vi "AlgorithmCentralGoal2Copy.vi"(0 "MatchBallX":dbl, 1 "MatchBallY":dbl, 2 "D1 X COM":dbl, 3 "D1Y COM":dbl, 4 "D2 X COM":dbl, 5 "D2 Y COM":dbl) -> (9 "LW":cluster{"kLW":dbl, "CoLW":dbl, "y":dbl, "y":dbl}, 11 "RW":cluster{"kRW":dbl, "CoRW":dbl, "y":dbl, "y":dbl}, 13 "output cluster":T1, 14 "Theta LG,LW":dbl, 15 "aRW":dbl, 16 "aS":dbl, 17 "min x":dbl, 18 "min x2":dbl, 19 "min x3":dbl)   [LabVIEW 2014]
panel:
  out "xD2BotS":dbl
  out "xD2ComS":dbl
  out "xD1BotS":dbl
  out "xD1ComS":dbl
  out "xD2BotR":dbl
  out "xD2ComR":dbl
  out "xD1BotR":dbl
  out "xD1ComR":dbl
  out "D2 X Bot fit 2":dbl
  out "D2 X Com fit":dbl
  out "D1 X Bot fit":dbl
  out "D1 X Com fit":dbl
  # "LOGIC"
  # "Left Goal"
  # "STRAIGHT"
  # "Left wall"
  # "Right Wall"
  # "Straight"
  # "sending data"
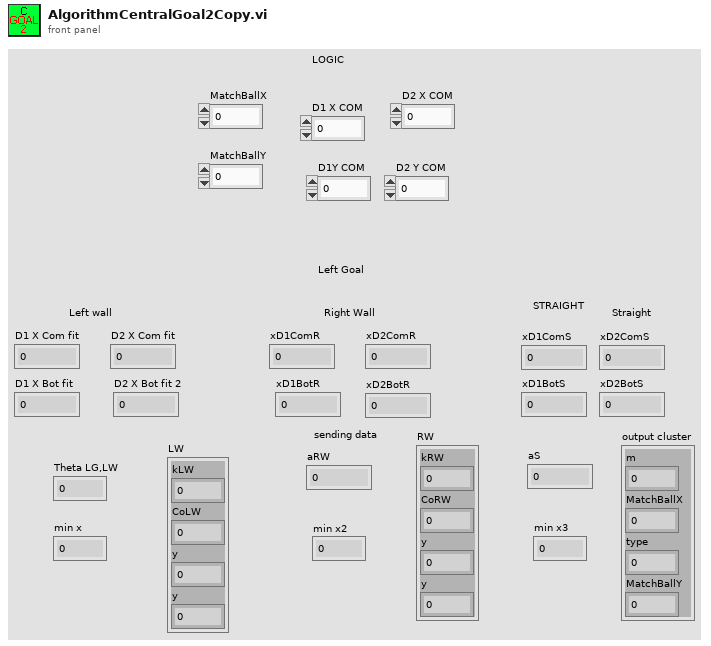
[diagram p1: front panel]
types:
  T1 = cluster{"m":dbl, "MatchBallX":dbl, "type":dbl, "MatchBallY":dbl}
  T2 = cluster{"m":dbl, "MatchBallX":dbl, "y":dbl, "MatchBallY":dbl}
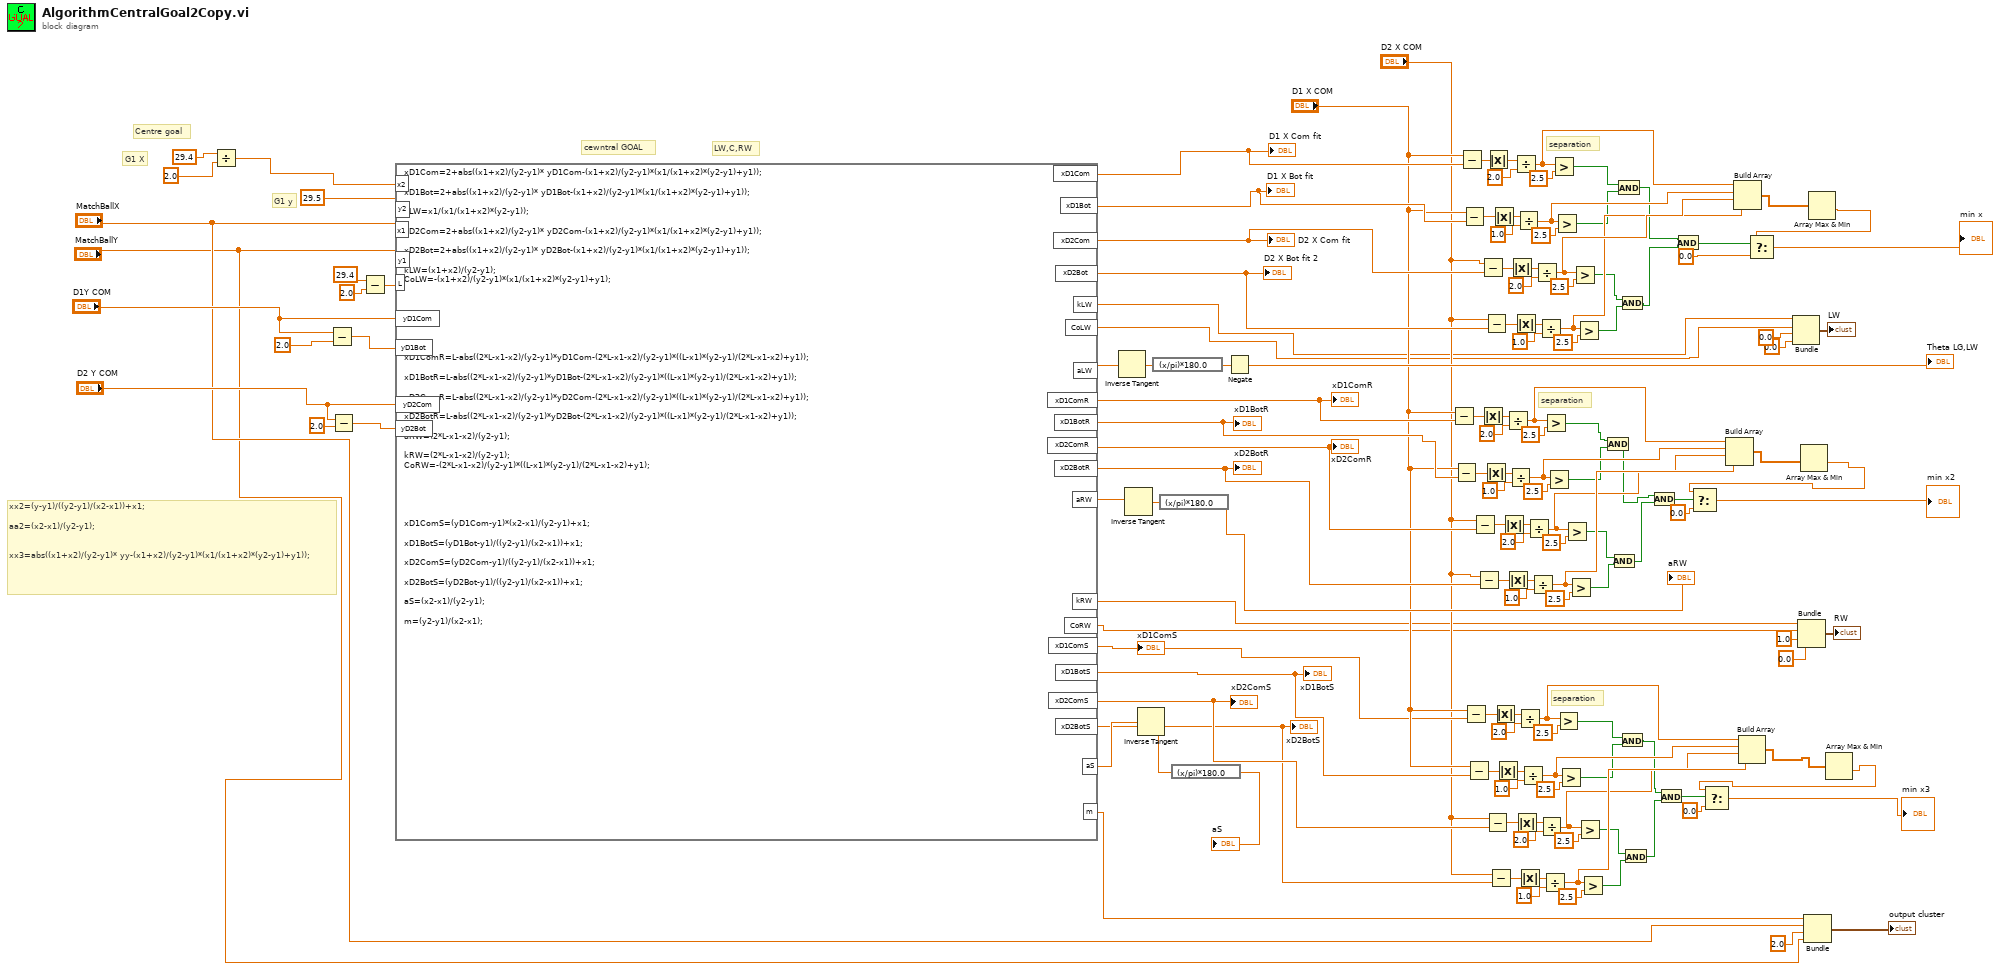
[diagram p0: block diagram]
diagram:
  # "Centre goal"
  # "G1 X"
  # "LW,C,RW"
  # "separation"
  # "separation"
  # "separation"
  # "cewntral GOAL"
  # "xx2=(y-y1)/((y2-y1)/(x2-x1))+x1;\n\naa2=(x2-x1)/(y2-y1);\n\n\nxx3=abs((x1+x2)/(y2-y1)* yy-(x1+x2)/(y2-y1)*(x1/(x1+x2)*(y2-y1)+y1));"
  # "G1 y"
  n1 = Divide(x=29.4, y=2.0) -> (x/y=w5:dbl)
  n2 = Subtract(x="D1Y COM", y=2.0) -> (x-y=w140:dbl)
  n3 = Subtract(x="D2 Y COM", y=2.0) -> (x-y=w135:dbl)
  n4 = Subtract(x=29.4 ("input variable"), y=2.0) -> (x-y=w20:dbl)
  n5 = formula code="xD1Com=2+abs((x1+x2)/(y2-y1)* yD1Com-(x1+x2)/(y2-y1)*(x1/(x1+x2)*(y2-y1)+y1));\n\nxD1Bot=2+abs((x1+x2)/(y2-y1)* yD1Bot-(x1+x2)/(y2-y1)*(x1/(x1+x2)*(y2-y1)+y1));\n\naLW=x1/(x1/(x1+x2)*(y2-y1));\n\nxD2Com=2+abs((x1+x2)/(y2-y1)* yD2Com-(x1+x2)/(y2-y1)*(x1/(x1+x2)*(y2-y1)+y1));\n\nxD2Bot=2+abs((x1+x2)/(y2-y1)* yD2Bot-(x1+x2)/(y2-y1)*(x1/(x1+x2)*(y2-y1)+y1));\n\nkLW=(x1+x2)/(y2-y1);\nCoLW=-(x1+x2)/(y2-y1)*(x1/(x1+x2)*(y2-y1)+y1);\n\n\n\n\n\n\n\nxD1ComR=L-abs((2*L-x1-x2)/(y2-y1)*yD1Com-(2*L-x1-x2)/(y2-y1)*((L-x1)*(y2-y1)/(2*L-x1-x2)+y1));\n\nxD1BotR=L-abs((2*L-x1-x2)/(y2-y1)*yD1Bot-(2*L-x1-x2)/(y2-y1)*((L-x1)*(y2-y1)/(2*L-x1-x2)+y1));\n\nxD2ComR=L-abs((2*L-x1-x2)/(y2-y1)*yD2Com-(2*L-x1-x2)/(y2-y1)*((L-x1)*(y2-y1)/(2*L-x1-x2)+y1));\n\nxD2BotR=L-abs((2*L-x1-x2)/(y2-y1)*yD2Bot-(2*L-x1-x2)/(y2-y1)*((L-x1)*(y2-y1)/(2*L-x1-x2)+y1));\n\naRW=(2*L-x1-x2)/(y2-y1);\n\nkRW=(2*L-x1-x2)/(y2-y1);\nCoRW=-(2*L-x1-x2)/(y2-y1)*((L-x1)*(y2-y1)/(2*L-x1-x2)+y1);\n\n\n\n\n\nxD1ComS=(yD1Com-y1)*(x2-x1)/(y2-y1)+x1;\n\nxD1BotS=(yD1Bot-y1)/((y2-y1)/(x2-x1))+x1;\n\nxD2ComS=(yD2Com-y1)/((y2-y1)/(x2-x1))+x1;\n\nxD2BotS=(yD2Bot-y1)/((y2-y1)/(x2-x1))+x1;\n\naS=(x2-x1)/(y2-y1);\n\nm=(y2-y1)/(x2-x1);"("x1"="MatchBallX", "x2"=w5, "y2"=29.5, "y1"="MatchBallY", "yD1Com"="D1Y COM", "yD2Com"="D2 Y COM", "yD1Bot"=w140, "yD2Bot"=w135, "L"=w20) -> ("xD1Com"=w128:dbl, "aLW"=w143:dbl, "xD1Bot"=w114:dbl, "xD2Com"=w119:dbl, "xD2Bot"=w109:dbl, "xD1ComR"=w82:dbl, "xD1BotR"=w81:dbl, "xD2ComR"=w80:dbl, "xD2BotR"=w79:dbl, "aRW"=w133:dbl, "xD1ComS"=w56:dbl, "aS"=w129:dbl, "xD1BotS"=w55:dbl, "xD2BotS"=w53:dbl, "xD2ComS"=w54:dbl, "kLW"=w18:dbl, "CoLW"=w17:dbl, "kRW"=w15:dbl, "CoRW"=w14:dbl, "m"=w12:dbl)
  "D1 X Com fit" <- w128
  "D1 X Bot fit" <- w114
  "D2 X Com fit" <- w119
  "D2 X Bot fit 2" <- w109
  "xD1ComR" <- w82
  "xD1BotR" <- w81
  "xD2ComR" <- w80
  "xD2BotR" <- w79
  "xD1ComS" <- w56
  "xD1BotS" <- w55
  "xD2ComS" <- w54
  "xD2BotS" <- w53
  n6 = Inverse Tangent(1:w143) -> (0:w144:dbl)
  n7 = Inverse Tangent(1:w133) -> (0:w134:dbl)
  n8 = Inverse Tangent(1:w129) -> (0:w130:dbl)
  n9 = expression code="(x/pi)*180.0" ("radians to degrees")(w144) -> (w141:dbl)
  n10 = expression code="(x/pi)*180.0" ("radians to degrees")(w134) -> (→"aRW":dbl)
  n11 = expression code="(x/pi)*180.0" ("radians to degrees")(w130) -> (→"aS":dbl)
  n12 = Negate(x=w141) -> (-x=→"Theta LG,LW":dbl)
  n13 = Subtract(x="D1 X COM", y=w82) -> (x-y=w83:dbl)
  n14 = Subtract(x="D1 X COM", y=w81) -> (x-y=w94:dbl)
  n15 = Subtract(x="D1 X COM", y=w128) -> (x-y=w127:dbl)
  n16 = Subtract(x="D1 X COM", y=w114) -> (x-y=w115:dbl)
  n17 = Subtract(x="D1 X COM", y=w56) -> (x-y=w58:dbl)
  n18 = Subtract(x="D1 X COM", y=w55) -> (x-y=w69:dbl)
  n19 = Subtract(x="D2 X COM", y=w80) -> (x-y=w90:dbl)
  n20 = Subtract(x="D2 X COM", y=w79) -> (x-y=w95:dbl)
  n21 = Subtract(x="D2 X COM", y=w119) -> (x-y=w120:dbl)
  n22 = Absolute Value(x=w83) -> (abs(x)=w84:dbl)
  n23 = Absolute Value(x=w94) -> (abs(x)=w93:dbl)
  n24 = Subtract(x="D2 X COM", y=w109) -> (x-y=w113:dbl)
  n25 = Subtract(x="D2 X COM", y=w54) -> (x-y=w65:dbl)
  n26 = Absolute Value(x=w127) -> (abs(x)=w126:dbl)
  n27 = Subtract(x="D2 X COM", y=w53) -> (x-y=w70:dbl)
  n28 = Absolute Value(x=w115) -> (abs(x)=w116:dbl)
  n29 = Absolute Value(x=w58) -> (abs(x)=w59:dbl)
  n30 = Absolute Value(x=w69) -> (abs(x)=w68:dbl)
  n31 = Absolute Value(x=w90) -> (abs(x)=w89:dbl)
  n32 = Divide(x=w84, y=2.0) -> (x/y=w100:dbl)
  n33 = Absolute Value(x=w95) -> (abs(x)=w96:dbl)
  n34 = Divide(x=w93, y=1.0) -> (x/y=w101:dbl)
  n35 = Absolute Value(x=w120) -> (abs(x)=w121:dbl)
  n36 = Divide(x=w126, y=2.0) -> (x/y=w107:dbl)
  n37 = Absolute Value(x=w113) -> (abs(x)=w112:dbl)
  n38 = Absolute Value(x=w65) -> (abs(x)=w64:dbl)
  n39 = Divide(x=w116, y=1.0) -> (x/y=w106:dbl)
  n40 = Divide(x=w59, y=2.0) -> (x/y=w75:dbl)
  n41 = Absolute Value(x=w70) -> (abs(x)=w71:dbl)
  n42 = Divide(x=w68, y=1.0) -> (x/y=w76:dbl)
  n43 = Divide(x=w89, y=2.0) -> (x/y=w102:dbl)
  n44 = Divide(x=w96, y=1.0) -> (x/y=w103:dbl)
  n45 = Divide(x=w121, y=2.0) -> (x/y=w105:dbl)
  n46 = Divide(x=w112, y=1.0) -> (x/y=w104:dbl)
  n47 = Divide(x=w64, y=2.0) -> (x/y=w77:dbl)
  n48 = Divide(x=w71, y=1.0) -> (x/y=w78:dbl)
  n49 = Greater?(x=w100, y=2.5) -> (0:w39:bool)
  n50 = Greater?(x=w101, y=2.5) -> (0:w38:bool)
  n51 = Greater?(x=w107, y=2.5) -> (0:w44:bool)
  n52 = Greater?(x=w106, y=2.5) -> (0:w43:bool)
  n53 = Greater?(x=w75, y=2.5) -> (0:w34:bool)
  n54 = Greater?(x=w76, y=2.5) -> (0:w33:bool)
  n55 = Greater?(x=w102, y=2.5) -> (0:w37:bool)
  n56 = Greater?(x=w103, y=2.5) -> (0:w36:bool)
  n57 = Greater?(x=w105, y=2.5) -> (0:w48:bool)
  n58 = Greater?(x=w104, y=2.5) -> (0:w47:bool)
  n59 = Greater?(x=w77, y=2.5) -> (0:w31:bool)
  n60 = Greater?(x=w78, y=2.5) -> (0:w30:bool)
  n61 = And(x=w39, y=w38) -> (x .and. y?=w40:bool)
  n62 = And(x=w37, y=w36) -> (x .and. y?=w35:bool)
  n63 = And(x=w44, y=w43) -> (x .and. y?=w42:bool)
  n64 = And(x=w48, y=w47) -> (x .and. y?=w45:bool)
  n65 = And(x=w34, y=w33) -> (x .and. y?=w32:bool)
  n66 = And(x=w31, y=w30) -> (x .and. y?=w29:bool)
  n67 = And(x=w40, y=w35) -> (x .and. y?=w41:bool)
  n68 = And(x=w32, y=w29) -> (x .and. y?=w28:bool)
  n69 = And(x=w42, y=w45) -> (x .and. y?=w46:bool)
  n70 = Build Array(w100, w101, w102, w103) -> (w25:dbl[])
  n71 = Build Array(w107, w106, w105, w104) -> (w27:dbl[])
  n72 = Build Array(w75, w76, w77, w78) -> (w23:dbl[])
  n73 = Bundle("kLW"=w18, "CoLW"=w17, "y"=0.0, "y"=0.0) -> (→"LW":cluster{"kLW":dbl, "CoLW":dbl, "y":dbl, "y":dbl})  [unwired: 1 in]
  n74 = Bundle("kRW"=w15, "CoRW"=w14, "y"=1.0, "y"=0.0) -> (→"RW":cluster{"kRW":dbl, "CoRW":dbl, "y":dbl, "y":dbl})  [unwired: 1 in]
  n75 = Array Max & Min(array=w25) -> (min value=w24:dbl)  [unwired: 3 out]
  n76 = Select(t=w24, s=w41, f=0.0 ("y")) -> (s? t:f=→"min x2":dbl)
  n77 = Bundle("m"=w12, "MatchBallX"="MatchBallX", "y"=2.0, "MatchBallY"="MatchBallY") -> (→"output cluster":T2)  [unwired: 1 in]
  n78 = Array Max & Min(array=w27) -> (min value=w26:dbl)  [unwired: 3 out]
  n79 = Select(t=w26, s=w46, f=0.0 ("y")) -> (s? t:f=→"min x":dbl)
  n80 = Array Max & Min(array=w23) -> (min value=w22:dbl)  [unwired: 3 out]
  n81 = Select(t=w22, s=w28, f=0.0 ("y")) -> (s? t:f=→"min x3":dbl)
